vi "sv_Fractional-octave Analysis with IC (linear mode).vi"(0 "scaled signal [EU]":dbl[](array[numeric]) format="%.2f", 1 "linear averaging mode":T1(ring), 2 "filter bank parameters":T2={"octave filter coefficients"=[{"filter structure"=enum."IIR 2nd Order", "Reverse Coefficients"=[1.0], "Forward Coefficients"=[]}], "lowpass filter coefficients"={"filter structure"=enum."IIR 2nd Order", "Reverse Coefficients"=[], "Forward Coefficients"=[]}, "number of samples to settle"=0, "number of decimation steps required"=[], "octave filter bandwidth"=[]}, 3 "internal filter state IN":T3, 4 "reset averaging (F)":bool, 5 "filter init/cont (init:F)":bool) -> (6 "linear avg band power [EU^2 rms]":dbl[](array[numeric]) format="%.2f", 7 "settled?":bool, 8 "internal filter state OUT":T3)   [LabVIEW 2017, in "SoundVib_Octave_2014 standard.lvlib"]
doc: "Performs a linear average fractional-octave analysis on the input signal. This VI requires the filter bank parameters and initialize filter state information the Design Octave Filter Set VI generates.\nThis VI returns the linear average power in each fractional-octave band.\nThe internal filter state IN and internal filter state OUT keep track of the internal state of the filter to ensure continuous operation of the filter. To achieve this continuous operation, you must call this VI the first time with filter init/cont set to FALSE. Call it all subsequent times with filter init/cont set to TRUE. Wire the internal filter state OUT of this call to the internal filter state IN for the next call to this VI."
uses:
  <vilib>/addons/Sound and Vibration/svt_Octave/SoundVib_Octave_2014 standard.lvlib
  <vilib>/addons/_NISVFA/_Shared subVIs/Controls/svc_Octave Filter State.ctl
  <vilib>/addons/_NISVFA/_Shared subVIs/Controls/svc_Octave Filter Bank Parameters.ctl
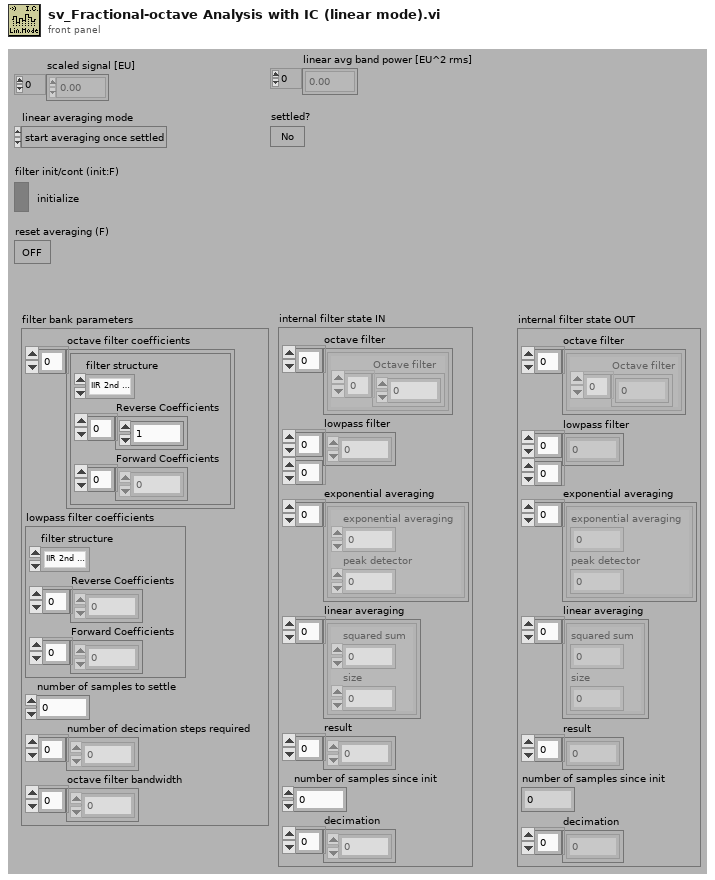
[diagram p1: front panel]
types:
  T1 = enum16{"start averaging once settled", "continuous averaging", "single averaging"}
  T2 = typedef "svc_Octave Filter Bank Parameters.ctl" = cluster{"octave filter coefficients":cluster{"filter structure":enum32{"IIR 2nd Order", "IIR 4th Order"}, "Reverse Coefficients":dbl[], "Forward Coefficients":dbl[]}[], "lowpass filter coefficients":cluster{"filter structure":enum32{"IIR 2nd Order", "IIR 4th Order"}, "Reverse Coefficients":dbl[], "Forward Coefficients":dbl[]}, "number of samples to settle":u64, "number of decimation steps required":i32[], "octave filter bandwidth":dbl[]}
  T3 = typedef "svc_Octave Filter State.ctl" = cluster{"octave filter":cluster{"Octave filter":dbl[]}[], "lowpass filter":dbl[][], "exponential averaging":cluster{"exponential averaging":dbl, "peak detector":dbl}[], "linear averaging":cluster{"squared sum":dbl, "size":dbl}[], "result":dbl[], "number of samples since init":u64, "decimation":dbl[]}
  T4 = enum16{"Linear", "Exponential", "Equal confidence", "Peak"}
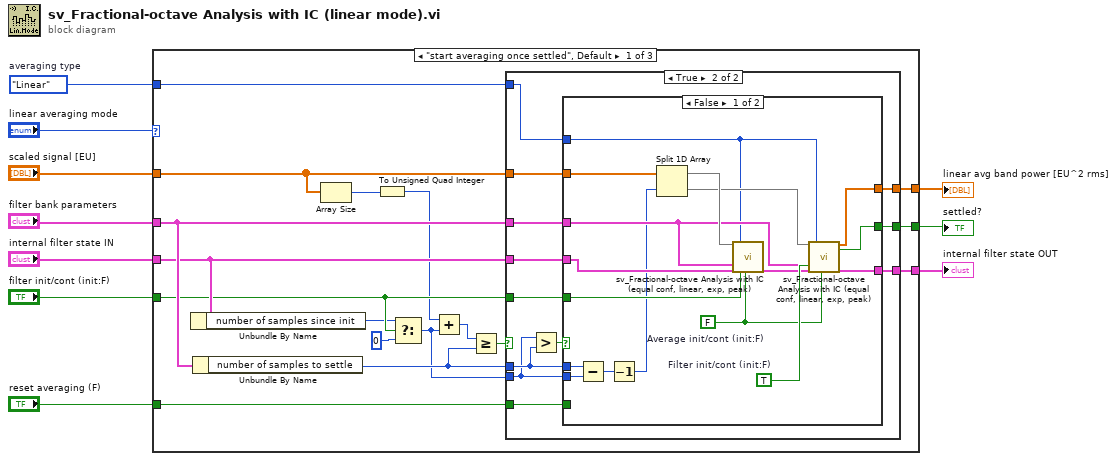
[diagram p0: block diagram]
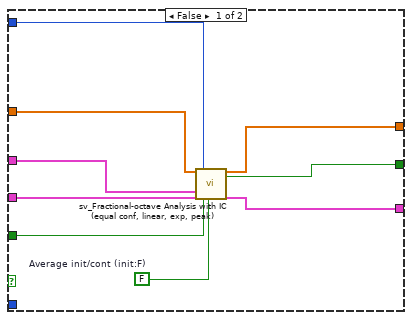
[diagram p2: hidden frame]
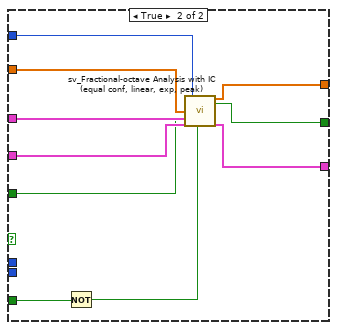
[diagram p3: hidden frame]
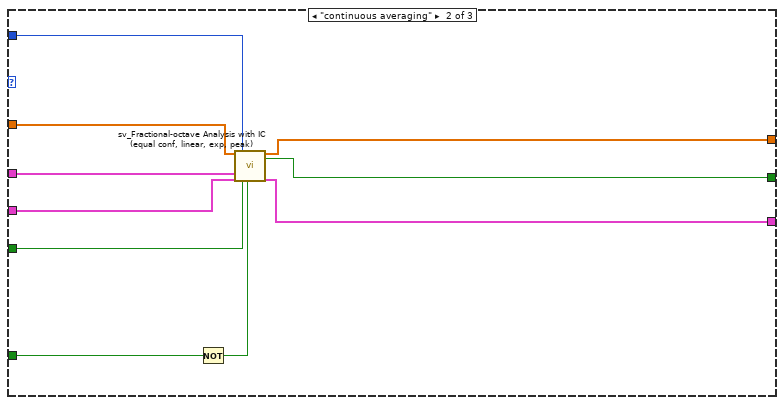
[diagram p4: hidden frame]
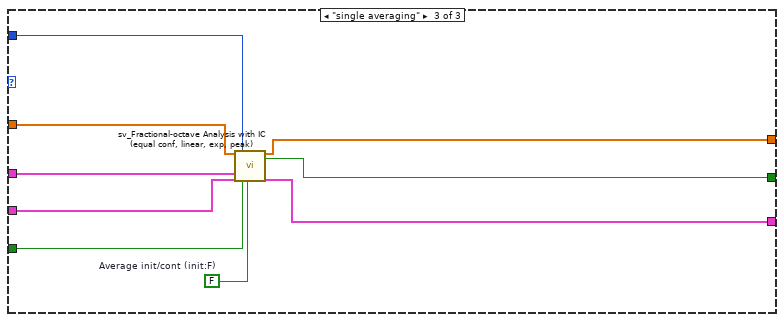
[diagram p5: hidden frame]
diagram:
  w10 = T4."Linear"  # averaging type
  n1 = case shown="\"start averaging once settled\", Default" "linear averaging mode" {
    tunnel: "scaled signal [EU]" -> [w21 w85 w94]
    tunnel: "filter bank parameters" -> [w27 w84 w93]
    tunnel: "internal filter state IN" -> [w26 w83 w92]
    tunnel: "filter init/cont (init:F)" -> [w23 w82 w91]
    tunnel: [w16 w81 w89] -> w7
    tunnel: [w15 w80 w88] -> w8
    tunnel: [w14 w79 w87] -> w9
    tunnel: "reset averaging (F)" -> [w13 w78 _]
    tunnel: w10 -> [w11 w76 w86]
    frame "start averaging once settled", Default {
      n2 = Unbundle By Name(w26) -> ("number of samples since init"=w22:u64)
      n3 = Unbundle By Name(w27) -> ("number of samples to settle"=w25:u64)
      n4 = Array Size(array=w21) -> (size(s)=w19:i32)
      n5 = To Unsigned Quad Integer(1:w19) -> (0:w12:u64)
      n6 = Select(t=w22, s=w23, f=u64 0) -> (s? t:f=w17:u64)
      n7 = Add(x=w12, y=w17) -> (x+y=w18:u64)
      n8 = Greater Or Equal?(x=w18, y=w25) -> (x >= y?=w24:bool)
      n9 = case shown="True" w24 {
        tunnel: w27 -> [w36 w48]
        tunnel: w21 -> [w35 w45]
        tunnel: w26 -> [w33 w47]
        tunnel: w23 -> [w32 w46]
        tunnel: w25 -> [_ w43]
        tunnel: w17 -> [_ w42]
        tunnel: [w31 w41] -> w16
        tunnel: [w30 w40] -> w15
        tunnel: [w29 w39] -> w14
        tunnel: w13 -> [_ w38]
        tunnel: w11 -> [w28 w37]
        frame False {
          w34 = FALSE  # Average init/cont (init:F)
          n10 = call <vilib>:"sv_Fractional-octave Analysis with IC (equal conf, linear, exp, peak).vi"("scaled signal [EU]"=w35, "filter bank parameters"=w36, "internal filter state IN"=w33, "averaging type"=w28, "filter init/cont (init:F)"=w32, "average init/cont (cont:T)"=w34) -> ("band power [EU^2 rms]"=w31:dbl[], "settled?"=w30:bool, "internal filter state OUT"=w29:T3)  [unwired: 9 in, 2 out]
        }
        frame True {
          n11 = Greater?(x=w42, y=w43) -> (0:w44:bool)
          n12 = case shown="False" w44 {
            tunnel: w48 -> [w55 w75]
            tunnel: w47 -> [w60 w74]
            tunnel: w46 -> [w59 w73]
            tunnel: w45 -> [w65 w72]
            tunnel: w43 -> [w64 _]
            tunnel: w42 -> [w63 _]
            tunnel: [w53 w71] -> w41
            tunnel: [w52 w70] -> w40
            tunnel: [w51 w69] -> w39
            tunnel: w38 -> [_ w68]
            tunnel: w37 -> [w49 w66]
            frame False {
              w58 = TRUE  # Filter init/cont (init:F)
              w54 = FALSE  # Average init/cont (init:F)
              n13 = Subtract(x=w64, y=w63) -> (x-y=w62:u64)
              n14 = Decrement(x=w62) -> (x-1=w50:u64)
              n15 = Split 1D Array(array=w65, index=w50) -> (first subarray=w61:dbl[], second subarray=w57:dbl[])
              n16 = call <vilib>:"sv_Fractional-octave Analysis with IC (equal conf, linear, exp, peak).vi"("scaled signal [EU]"=w61, "filter bank parameters"=w55, "internal filter state IN"=w60, "averaging type"=w49, "filter init/cont (init:F)"=w59, "average init/cont (cont:T)"=w54) -> ("internal filter state OUT"=w56:T3)  [unwired: 9 in, 4 out]
              n17 = call <vilib>:"sv_Fractional-octave Analysis with IC (equal conf, linear, exp, peak).vi"("scaled signal [EU]"=w57, "filter bank parameters"=w55, "internal filter state IN"=w56, "averaging type"=w49, "filter init/cont (init:F)"=w58, "average init/cont (cont:T)"=w54) -> ("band power [EU^2 rms]"=w53:dbl[], "settled?"=w52:bool, "internal filter state OUT"=w51:T3)  [unwired: 9 in, 2 out]
            }
            frame True {
              n18 = Not(x=w68) -> (.not. x?=w67:bool)
              n19 = call <vilib>:"sv_Fractional-octave Analysis with IC (equal conf, linear, exp, peak).vi"("scaled signal [EU]"=w72, "filter bank parameters"=w75, "internal filter state IN"=w74, "averaging type"=w66, "filter init/cont (init:F)"=w73, "average init/cont (cont:T)"=w67) -> ("band power [EU^2 rms]"=w71:dbl[], "settled?"=w70:bool, "internal filter state OUT"=w69:T3)  [unwired: 9 in, 2 out]
            }
          }
        }
      }
    }
    frame "continuous averaging" {
      n20 = Not(x=w78) -> (.not. x?=w77:bool)
      n21 = call <vilib>:"sv_Fractional-octave Analysis with IC (equal conf, linear, exp, peak).vi"("scaled signal [EU]"=w85, "filter bank parameters"=w84, "internal filter state IN"=w83, "averaging type"=w76, "filter init/cont (init:F)"=w82, "average init/cont (cont:T)"=w77) -> ("band power [EU^2 rms]"=w81:dbl[], "settled?"=w80:bool, "internal filter state OUT"=w79:T3)  [unwired: 9 in, 2 out]
    }
    frame "single averaging" {
      w90 = FALSE  # Average init/cont (init:F)
      n22 = call <vilib>:"sv_Fractional-octave Analysis with IC (equal conf, linear, exp, peak).vi"("scaled signal [EU]"=w94, "filter bank parameters"=w93, "internal filter state IN"=w92, "averaging type"=w86, "filter init/cont (init:F)"=w91, "average init/cont (cont:T)"=w90) -> ("band power [EU^2 rms]"=w89:dbl[], "settled?"=w88:bool, "internal filter state OUT"=w87:T3)  [unwired: 9 in, 2 out]
    }
  }
  "linear avg band power [EU^2 rms]" <- w7
  "internal filter state OUT" <- w9
  "settled?" <- w8
